vi "MoveXY.vi"(4 "Reset Position (F)":bool, 5 "Step Type (Half Step)":T1(ring), 6 "Standby at end (No Change)":enum16{"FALSE", "TRUE", "No Change"}(ring)=enum."No Change", 7 "Hold at end (No Change)":enum16{"FALSE", "TRUE", "No Change"}(ring)=enum."No Change", 8 "error in (no error)":errorcluster, 9 "Step Rate (ms)":u16, 10 "Delta Position\n(Steps|HalfSteps)":i32, 11 "Motor":u8=1 min=1 max=6 step=1) -> (0 "error out":errorcluster, 1 "Final Position (Half Steps)":i32, 2 "Switch":bool, 3 "Error descriptions":T2)   [LabVIEW 2014]
doc: "A VI to move the motors of the Arrick controller (e.g., the XY table). Basic operation is to move a motor (#1--6) by a certain number of steps. The motors controlled by LPT1 are normally #3 and #4. Speed is determined by the time between steps.\n\nA \"step\" is actually a whole or half step, as described in the controller manual. Motors may be left engaged (\"Hold\") at either full or half (\"Standby\") power, or not held at all. This should be specified on the first call, but subsequent calls may use the default of No Change. Note that Hold and Standby apply to _pairs_ of motors (e.g., 3 & 4).\n\nAbsolute position (in half-steps) is maintained internally, starting with 0 when subVI is first loaded into memory. Resetting the position counter to zero occurs before any motion. If other subVIs move the motors, these positions will become incorrect. The other output indicates the state of the limit switch at the end of execution. Note that this subVI attempts motion regardless of switch status.\n\nErrors returned are specific to this subVI. The Error Description output can be unbundled for use with the General Error Hander node to produce human-readable error messages."
uses:
  <vilib>/Platform/portaccess.llb/In Port8.vi
  <vilib>/Platform/portaccess.llb/Out Port8.vi
panel:
  out "Positions":i32[](array[numeric])
  out "Standby":bool caption="(on=high=standby)"
  out "Enabled":bool caption="(on=low=enabled)"
  # "INPUTS"
  # "MOTOR STATES"
  # "OUTPUTS"
  # "WARNING!\nStandby and Hold states apply to BOTH motors on a given port.  Hold means that motor is left with power holding it in position.  Standby means that a hold is only 1/2 power."
  # "This subVI uses this array (which is not wired to the connector block) as internal memory to keep track of the motor positions.  The state will be remembered as long as LabVIEW keeps the subVI loaded in memory."
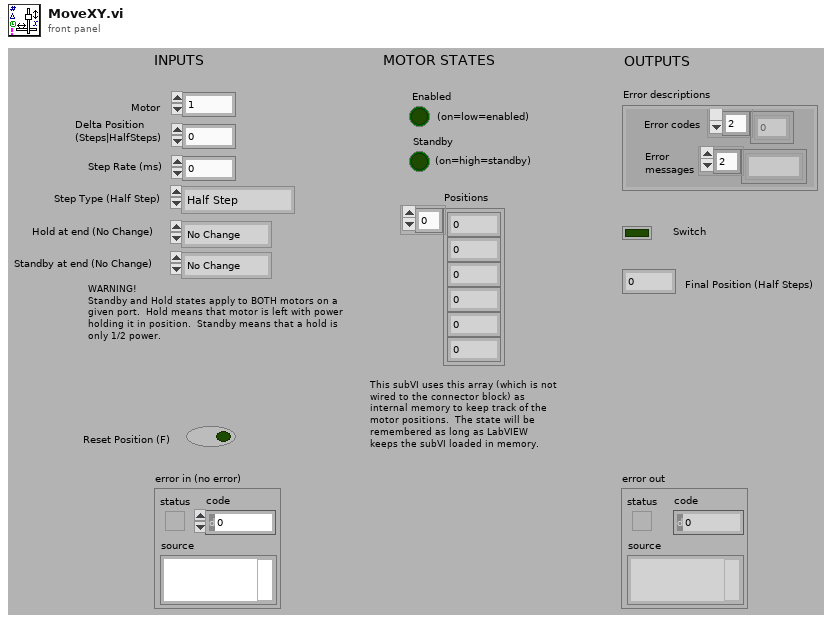
[diagram p1: front panel]
types:
  T1 = enum16{"Half Step", "Full-Single Step", "Full-Double Step"}
  T2 = cluster{"Error codes":i32[], "Error\nmessages":string[]}
  T3 = cluster{"[0]":bool, "[1]":bool, "[2]":bool, "[3]":bool, "[4]":bool, "[5]":bool, "[6]":bool, "[7]":bool}
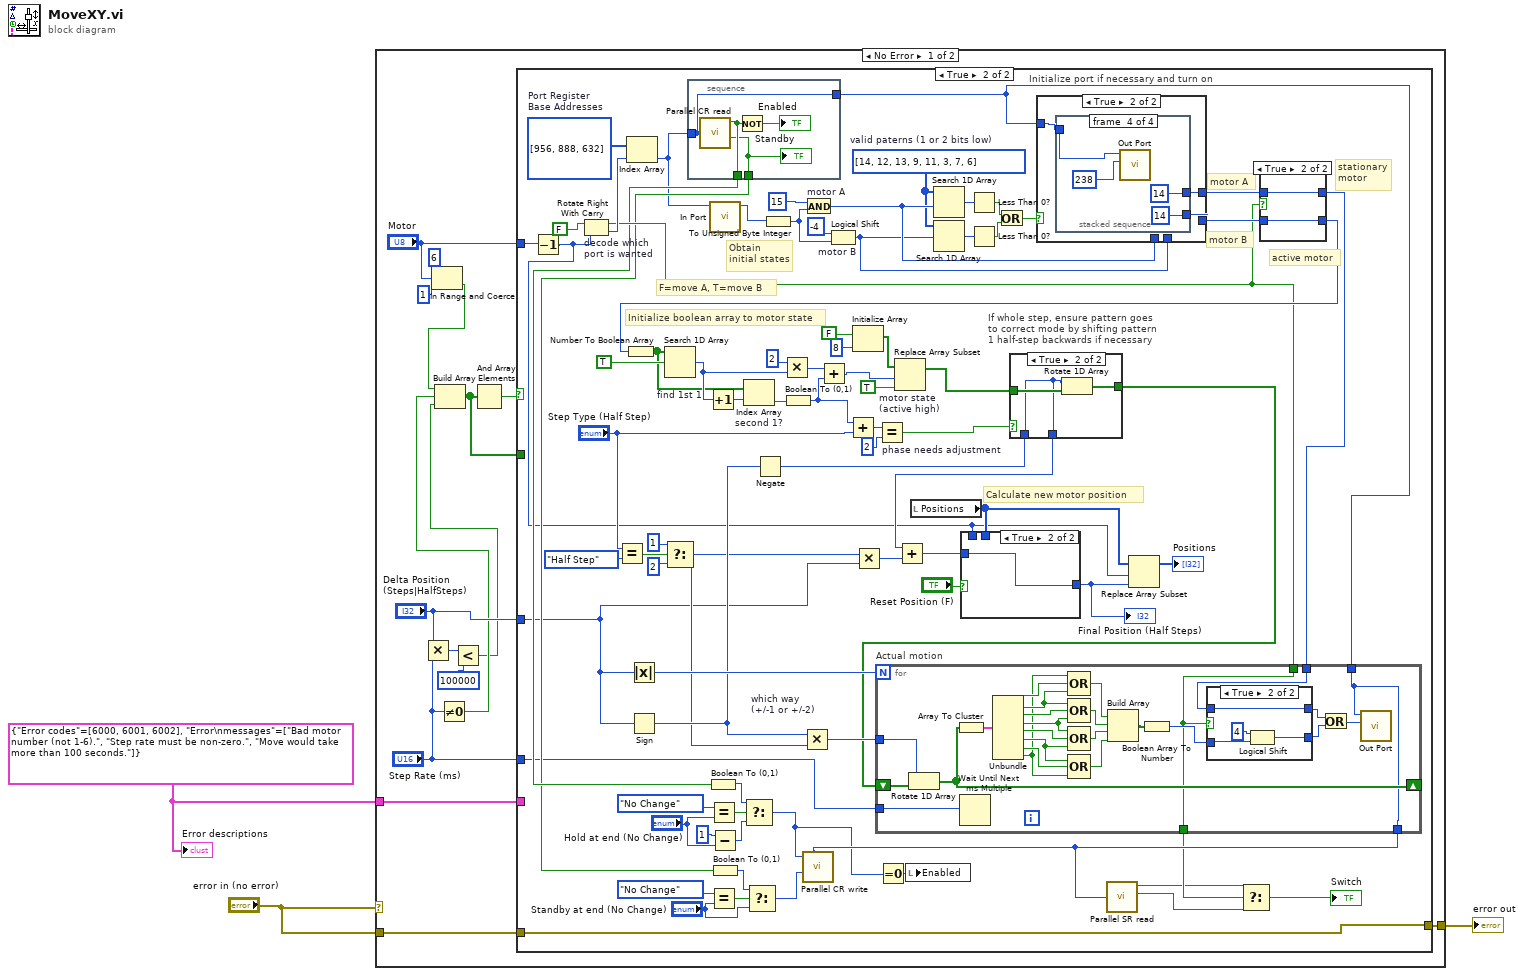
[diagram p0: block diagram]
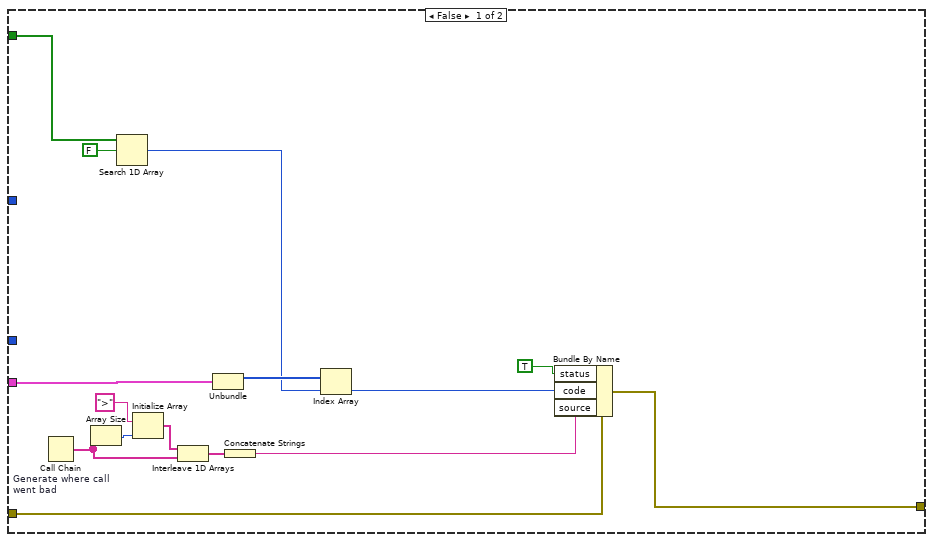
[diagram p2: hidden frame]
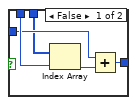
[diagram p3: hidden frame]
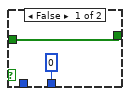
[diagram p5: hidden frame]
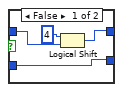
[diagram p6: hidden frame]
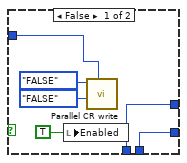
[diagram p7: hidden frame]
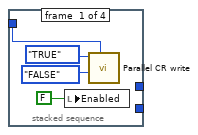
[diagram p8: hidden frame]
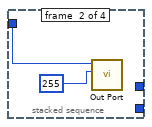
[diagram p9: hidden frame]
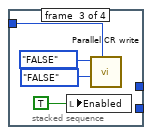
[diagram p10: hidden frame]
diagram:
  w2 = T2 {"Error codes"=[6000, 6001, 6002], "Error\nmessages"=["Bad motor number (not 1-6).", "Step rate must be non-zero.", "Move would take more than 100 seconds."]} ("Error descriptions")
  n1 = case shown="No Error" "error in (no error)" {
    tunnel: "error in (no error)" -> [w15 w191]
    tunnel: [w16 w191] -> w3
    tunnel: w2 -> [w13 _]
    frame No Error {
      n2 = Multiply(x="Delta Position\n(Steps|HalfSteps)", y="Step Rate (ms)") -> (x*y=w10:i32)
      n3 = In Range and Coerce(upper limit=u8 6, x="Motor", lower limit=u8 1) -> (In Range?=w7:bool)  [unwired: 1 out]
      n4 = Not Equal To 0?(x="Step Rate (ms)") -> (x != 0?=w6:bool)
      n5 = Less?(x=w10, y=100000) -> (x < y?=w5:bool)
      n6 = Build Array(w7, w6, w5) -> (w4:bool[])
      n7 = And Array Elements(Boolean array=w4) -> (logical AND=w8:bool)
      n8 = case shown="True" w8 {
        tunnel: "Motor" -> [_ w91]
        tunnel: [w24 w92] -> w16
        tunnel: w15 -> [w25 w92]
        tunnel: "Step Rate (ms)" -> [_ w45]
        tunnel: w13 -> [w23 _]
        tunnel: "Delta Position\n(Steps|HalfSteps)" -> [_ w44]
        tunnel: w4 -> [w19 _]
        frame False {
          n9 = Call Chain "Generate where call went bad"() -> (call chain=w28:string[])
          n10 = Array Size(array=w28) -> (size(s)=w32:i32)
          n11 = Search 1D Array(1D array=w19, element=FALSE) -> (index of element=w21:i32)  [unwired: 1 in]
          n12 = Initialize Array(">", w32) -> (w29:string[])
          n13 = Interleave 1D Arrays(w29, w28) -> (w30:string[])
          n14 = Unbundle(w23) -> ("Error codes"=w22:i32[])  [unwired: 1 out]
          n15 = Concatenate Strings(w30) -> (w26:string)
          n16 = Index Array(array=w22, index=w21) -> (element=w20:i32)
          n17 = Bundle By Name(cluster=w25, "status"=TRUE, "code"=w20, "source"=w26) -> (w24:errorcluster)
        }
        frame True {
          w36 = i32[] [14, 12, 13, 9, 11, 3, 7, 6]  # valid paterns (1 or 2 bits low)
          w113 = u32[] [956, 888, 632]  # Port Register Base Addresses
          # "Calculate new motor position"
          # "F=move A, T=move B"
          # "stationary\nmotor"
          # "active motor"
          # "motor B"
          # "motor A"
          # "Initialize boolean array to motor state"
          # "Obtain\ninitial states"
          n18 = Decrement(x=w91) -> (x-1=w48:u8)
          n19 = Rotate Right With Carry "decode which\nport is wanted"(2:w48, 3:FALSE ("carry")) -> (0:w114:u8, 1:w70:bool)
          n20 = Equal?(x="Step Type (Half Step)", y=T1."Half Step") -> (x = y?=w84:bool)
          n21 = Index Array(array=w113, index=w114) -> (element=w34:u32)
          n22 = Absolute Value(x=w44) -> (abs(x)=w83:i32)
          n23 = Sign(1:w44) -> (0:w62:i32)
          n24 = Select(t=1, s=w84, f=2) -> (s? t:f=w46:i32)
          n25 = stacked-sequence {
            tunnel: w34 -> [w125]
            tunnel: [w125] -> w59
            tunnel: [w124] -> w61
            tunnel: [w123] -> w60
            frame #0 {
              n26 = call "Parallel CR read.vi"("Port Base Address"=w125) -> ("-Strobe"=w124:bool, "-Init"=w123:bool)  [unwired: 2 out]
              "Standby" <- w123
              n27 = Not(x=w124) -> (.not. x?=→"Enabled":bool)
            }
          }
          n28 = Boolean To (0,1)(Boolean=w61) -> (0, 1=w58:i16)
          n29 = Equal?(x=enum16{"FALSE", "TRUE", "No Change"}."No Change", y="Hold at end (No Change)") -> (x = y?=w69:bool)
          n30 = Equal?(x=enum16{"FALSE", "TRUE", "No Change"}."No Change", y="Standby at end (No Change)") -> (x = y?=w68:bool)
          n31 = call-poly <vilib>:"In Port.vi"("address"=w34) -> ("data read"=w35:i8)  [unwired: 7 in, 1 out]
          n32 = Subtract(x=1, y="Hold at end (No Change)") -> (x-y=w65:i32)
          n33 = Boolean To (0,1)(Boolean=w60) -> (0, 1=w57:i16)
          n34 = Select(t=w58, s=w69, f=w65) -> (s? t:f=w37:i32)
          n35 = Select(t=w57, s=w68, f="Standby at end (No Change)") -> (s? t:f=w66:u16)
          n36 = Negate(x=w62) -> (-x=w76:i32)
          n37 = To Unsigned Byte Integer(number=w35) -> (unsigned 8bit integer=w105:u8)
          n38 = Multiply "which way\n(+/-1 or +/-2)"(x=w62, y=w46) -> (x*y=w80:i32)
          n39 = And "motor A"(x=u8 15, y=w105) -> (x .and. y?=w90:u8)
          n40 = Logical Shift "motor B"(y=i16 -4, x=w105) -> (x << y=w89:u8)
          n41 = Initialize Array(FALSE, 8 ("dimension size")) -> (w102:bool[])
          n42 = Multiply(x=w46, y=w44) -> (x*y=w52:i32)
          n43 = Equal To 0?(x=w37) -> (x = 0?=w38:bool)
          n44 = local write "Enabled"(w38) -> ()
          n45 = local read "Positions"() -> (w50:i32[])
          n46 = Search 1D Array(1D array=w36, element=w90) -> (index of element=w110:i32)  [unwired: 1 in]
          n47 = Search 1D Array(1D array=w36, element=w89) -> (index of element=w109:i32)  [unwired: 1 in]
          n48 = Less Than 0?(x=w110) -> (x < 0?=w108:bool)
          n49 = Less Than 0?(x=w109) -> (x < 0?=w107:bool)
          n50 = Or(x=w108, y=w107) -> (x .or. y?=w106:bool)
          n51 = case "Initialize port if necessary and turn on" shown="True" w106 {
            tunnel: w59 -> [w171 w176]
            tunnel: [w173 w175] -> w74
            tunnel: [w172 w174] -> w73
            tunnel: w90 -> [w173 _]
            tunnel: w89 -> [w172 _]
            frame False {
              n52 = local write "Enabled"(TRUE) -> ()
              n53 = call "Parallel CR write.vi"("-Strobe"=enum16{"FALSE", "TRUE", "No Change"}."FALSE", "-Init"=enum16{"FALSE", "TRUE", "No Change"}."FALSE", "Port Base Address"=w171) -> ()  [unwired: 2 in, 1 out]
            }
            frame True {
              n54 = stacked-sequence {
                tunnel: w176 -> [w180 w182 w186 w188]
                tunnel: [_ _ _ u8 14 ("value")] -> w175
                tunnel: [_ _ _ u8 14 ("value")] -> w174
                frame #0 {
                  n55 = local write "Enabled"(FALSE) -> ()
                  n56 = call "Parallel CR write.vi"("-Strobe"=enum16{"FALSE", "TRUE", "No Change"}."TRUE", "-Init"=enum16{"FALSE", "TRUE", "No Change"}."FALSE", "Port Base Address"=w180) -> ()  [unwired: 2 in, 1 out]
                }
                frame #1 {
                  n57 = call-poly <vilib>:"Out Port.vi"("write value"=u8 255 ("value"), "address"=w182) -> ()  [unwired: 7 in, 1 out]
                }
                frame #2 {
                  n58 = local write "Enabled"(TRUE) -> ()
                  n59 = call "Parallel CR write.vi"("-Strobe"=enum16{"FALSE", "TRUE", "No Change"}."FALSE", "-Init"=enum16{"FALSE", "TRUE", "No Change"}."FALSE", "Port Base Address"=w186) -> ()  [unwired: 2 in, 1 out]
                }
                frame #3 {
                  n60 = call-poly <vilib>:"Out Port.vi"("write value"=u8 238 ("value"), "address"=w188) -> ()  [unwired: 7 in, 1 out]
                }
              }
            }
          }
          n61 = case shown="True" w70 {
            tunnel: [w126 w129] -> w71
            tunnel: w74 -> [w127 w129]
            tunnel: [w127 w128] -> w72
            tunnel: w73 -> [w126 w128]
            frame False {
            }
            frame True {
            }
          }
          n62 = Number To Boolean Array(number=w72) -> (Boolean array=w97:bool[])
          n63 = Search 1D Array "find 1st 1"(1D array=w97, element=TRUE) -> (index of element=w99:i32)  [unwired: 1 in]
          n64 = Increment(x=w99) -> (x+1=w98:i32)
          n65 = Index Array "second 1?"(array=w97, index=w98) -> (element=w96:bool)
          n66 = Multiply(x=2 ("n"), y=w99) -> (x*y=w95:i32)
          n67 = Boolean To (0,1)(Boolean=w96) -> (0, 1=w88:i16)
          n68 = Add(x=w95, y=w88) -> (x+y=w93:i32)
          n69 = Add(x=w88, y="Step Type (Half Step)") -> (x+y=w79:u16)
          n70 = Equal? "phase needs adjustment"(x=w79, y=u16 2 ("x")) -> (x = y?=w87:bool)
          n71 = Replace Array Subset "motor state\n(active high)"(array=w102, new element=TRUE ("new element/subarray"), index=w93) -> (w77:bool[])
          n72 = case "If whole step, ensure pattern goes\nto correct mode by shifting pattern\n1 half-step backwards if necessary" shown="True" w87 {
            tunnel: w77 -> [w131 w134]
            tunnel: w76 -> [_ w132]
            tunnel: [w131 w133] -> w75
            tunnel: [0 w132] -> w51
            frame False {
            }
            frame True {
              n73 = Rotate 1D Array(1:w134, 2:w132) -> (0:w133:bool[])
            }
          }
          n74 = for "Actual motion" {
            N: w83 -> [_]
            shift-right: [w145] -> _
            shift-left: w75 -> [w155]
            tunnel: w80 -> [w144]
            tunnel: w71 -> [w142]
            tunnel: w70 -> [w137]
            tunnel: w59 -> [w135]
            tunnel: [w135] -> w43
            tunnel: w45 -> [w138]
            tunnel: [w137] -> w42
            n75 = Rotate 1D Array(1:w155, 2:w144) -> (0:w145:bool[])
            n76 = Array To Cluster(array=w145) -> (cluster=w159:T3)
            n77 = Wait Until Next ms Multiple(millisecond multiple=w138) -> ()  [unwired: 1 out]
            n78 = Unbundle(w159) -> ("[0]"=w158:bool, "[1]"=w154:bool, "[2]"=w157:bool, "[3]"=w153:bool, "[4]"=w156:bool, "[5]"=w152:bool, "[6]"=w151:bool, "[7]"=w150:bool)
            n79 = Compound Arithmetic op=OR(w150, w158, w154) -> (w147:bool)
            n80 = Compound Arithmetic op=OR(w154, w157, w153) -> (w149:bool)
            n81 = Compound Arithmetic op=OR(w153, w156, w152) -> (w148:bool)
            n82 = Compound Arithmetic op=OR(w152, w151, w150) -> (w146:bool)
            n83 = Build Array(w147, w149, w148, w146) -> (w143:bool[])
            n84 = Boolean Array To Number(Boolean array=w143) -> (number=w141:u32)
            n85 = case shown="True" w137 {
              tunnel: w142 -> [w161 w164]
              tunnel: w141 -> [w162 w166]
              tunnel: [w162 w165] -> w139
              tunnel: [w160 w164] -> w140
              frame False {
                n86 = Logical Shift(y=i16 4, x=w161) -> (x << y=w160:u8)
              }
              frame True {
                n87 = Logical Shift(y=i16 4, x=w166) -> (x << y=w165:u32)
              }
            }
            n88 = Or(x=w140, y=w139) -> (x .or. y?=w136:u32)
            n89 = call-poly <vilib>:"Out Port.vi"("write value"=w136, "address"=w135) -> ()  [unwired: 7 in, 1 out]
          }
          n90 = call "Parallel CR write.vi"("-Strobe"=w37, "-Init"=w66, "Port Base Address"=w43) -> ()  [unwired: 2 in, 1 out]
          n91 = Add(x=w51, y=w52) -> (x+y=w53:i32)
          n92 = case shown="True" "Reset Position (F)" {
            tunnel: w48 -> [w120 _]
            tunnel: w53 -> [w118 w121]
            tunnel: [w117 w121] -> w47
            tunnel: w50 -> [w116 _]
            frame False {
              n93 = Index Array(array=w116, index=w120) -> (element=w119:i32)
              n94 = Add(x=w118, y=w119) -> (x+y=w117:i32)
            }
            frame True {
            }
          }
          "Final Position (Half Steps)" <- w47
          n95 = call "Parallel SR read.vi"("Port Base Address"=w43) -> ("Paper Empty"=w40:bool, "Select"=w41:bool)  [unwired: 3 out]
          n96 = Replace Array Subset(array=w50, new element=w47, index=w48) -> (→"Positions":i32[])
          n97 = Select(t=w41, s=w42, f=w40) -> (s? t:f=→"Switch":bool)
        }
      }
    }
    frame Error {
    }
  }
  "error out" <- w3
  "Error descriptions" <- w2
